vi "Read Configuration.vi"(8 "error in (no error)":errorcluster, 11 "Configuration File Path":path) -> (0 "error out":errorcluster, 3 "Ports to Check":T1)   [LabVIEW 2019]
doc: "Reads configuration file and returns ports to check."
uses:
  controls/Ports to Check.ctl
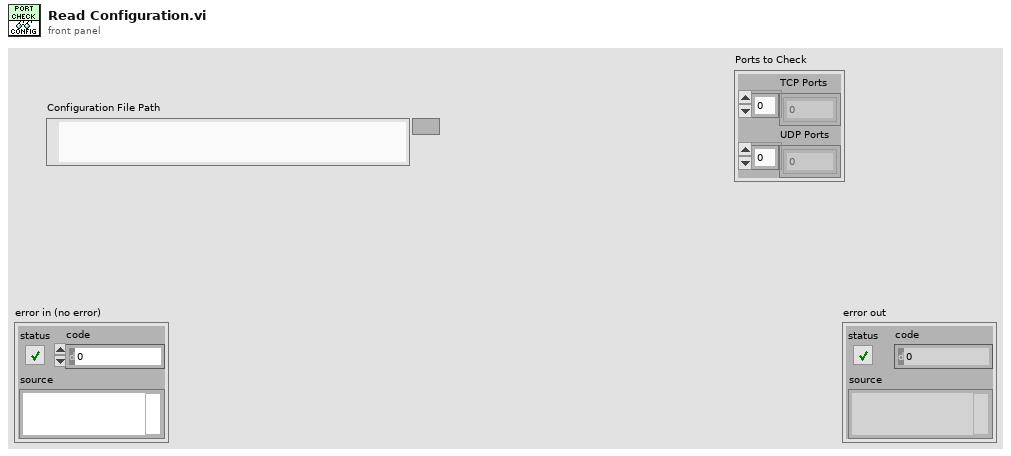
[diagram p1: front panel]
types:
  T1 = typedef "Ports to Check.ctl" = cluster{"TCP Ports":u16[], "UDP Ports":u16[]}
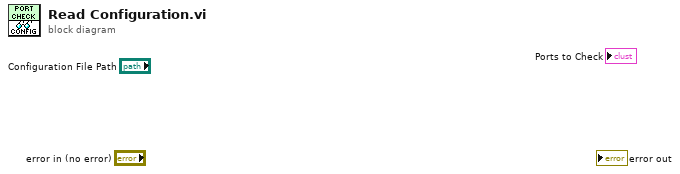
[diagram p0: block diagram]
diagram:
